vi "Flush Spy Queue.vi"(8 "error in (no error)":errorcluster, 11 "Mock Log Handler in":refnum<class "Mock Log Handler.lvclass">) -> (0 "error out":errorcluster, 3 "Mock Log Handler out":refnum<class "Mock Log Handler.lvclass">)   [LabVIEW 2020, in "Mock Log Handler.lvclass"]
uses:
  Mock Log Handler.lvclass
  Mock Log Handler.lvclass/Mock Log Handler.ctl
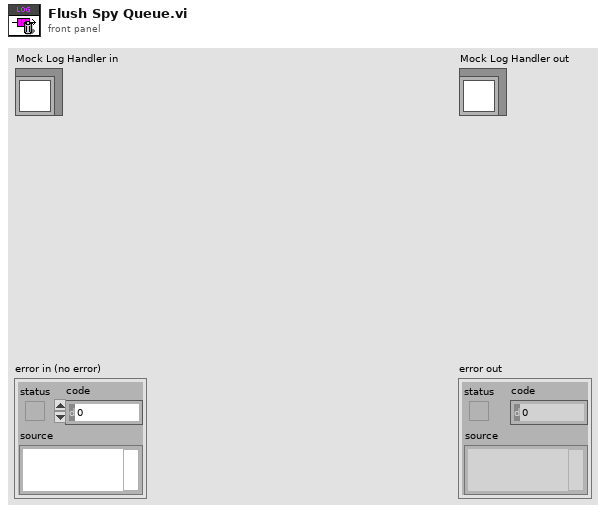
[diagram p1: front panel]
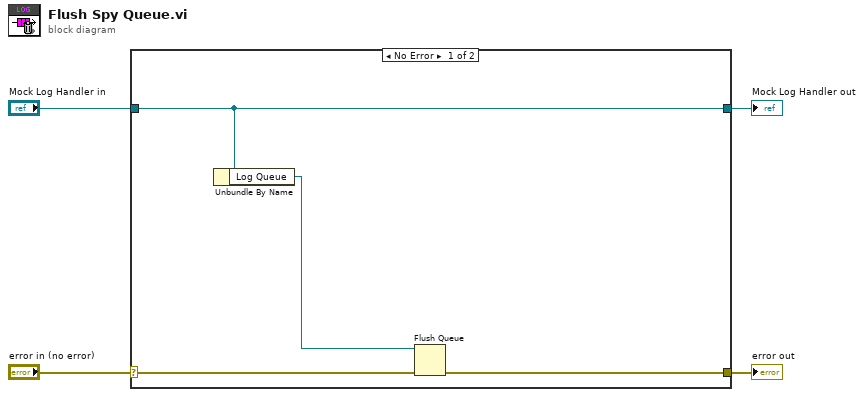
[diagram p0: block diagram]
diagram:
  n1 = case shown="No Error" "error in (no error)" {
    selector: "error in (no error)" -> [w8 w10]
    tunnel: [w6 w10] -> w3
    tunnel: [w7 w9] -> w1
    tunnel: "Mock Log Handler in" -> [w7 w9]
    frame No Error {
      n2 = Unbundle By Name(w7) -> ("Log Queue"=w5:refnum<queue>)
      n3 = Flush Queue(queue=w5, error in (no error)=w8) -> (error out=w6:errorcluster)  [unwired: 2 out]
    }
    frame Error {
    }
  }
  "error out" <- w3
  "Mock Log Handler out" <- w1
